vi "Read Map.vi"(8 "error in (no error)":errorcluster, 11 "Remap Bus in":refnum<class "Alias Bus.lvclass">) -> (0 "error out":errorcluster, 2 "Map":T1, 3 "Remap Bus out":refnum<class "Alias Bus.lvclass">)   [LabVIEW 2021, in "Alias Bus.lvclass"]
uses:
  Alias Bus.lvclass
  Support/Remap Type.ctl
  Alias Bus.lvclass/Alias Bus.ctl
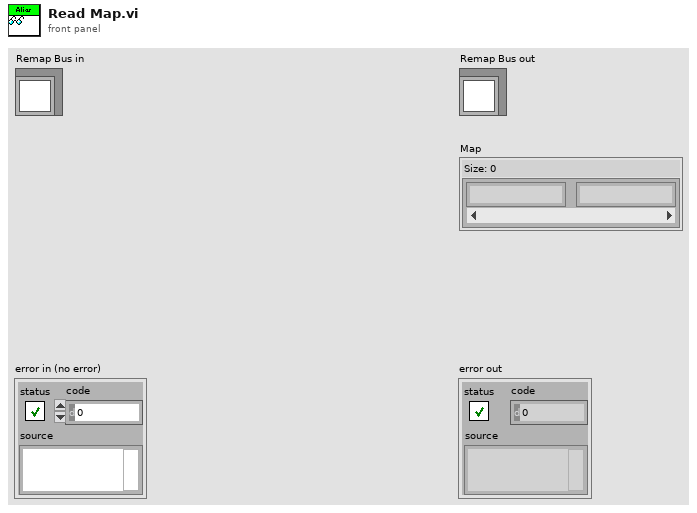
[diagram p1: front panel]
types:
  T1 = typedef "Alias Bus.lvclass/Remap Type.ctl" = map{string, string}
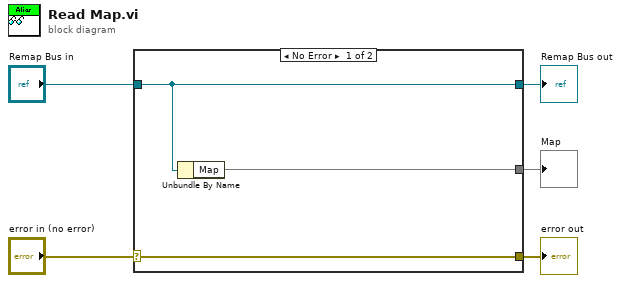
[diagram p0: block diagram]
diagram:
  n1 = case shown="No Error" "error in (no error)" {
    selector: "error in (no error)" -> [w8 w9]
    tunnel: [w8 w9] -> w4
    tunnel: [w7 w10] -> w2
    tunnel: "Remap Bus in" -> [w7 w10]
    tunnel: [w6 _] -> w1
    frame No Error {
      n2 = Unbundle By Name(w7) -> ("Map"=w6:T1)
    }
    frame Error {
    }
  }
  "error out" <- w4
  "Remap Bus out" <- w2
  "Map" <- w1
